vi "String to I16_2.vi"(11 "Test Case In":refnum<class "test Electronic Datasheet.lvclass">) -> (0 "error out":errorcluster, 3 "Test Case Out":refnum<class "test Electronic Datasheet.lvclass">)   [LabVIEW 2024, in "test Electronic Datasheet.lvclass"]
uses:
  test Electronic Datasheet.lvclass
  test Electronic Datasheet.lvclass/test Electronic Datasheet.ctl
  Core/Electronic Datasheet.lvlib
  d54f7c7f-f69a-4a4c-9201-5aaad2364e05.vi
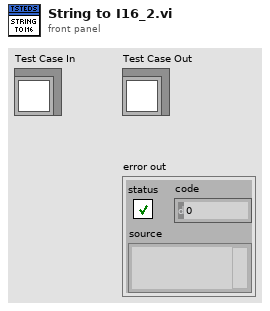
[diagram p1: front panel]
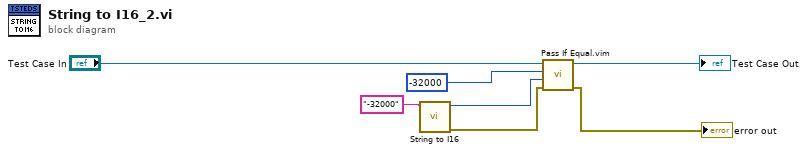
[diagram p0: block diagram]
diagram:
  n1 = call "String to I16.vi"("String"="-32000") -> ("error out"=w3:errorcluster, "I16"=w1:i16)  [unwired: 9 in]
  n2 = call "Pass If Equal.vim"("error in (no error)"=w3, "Actual"=w1, "Expected"=i16 -32000, "LUnit Test Case In"="Test Case In") -> ("error out"=→"error out":errorcluster, "LUnit Test Case Out"=→"Test Case Out":refnum<class "test Electronic Datasheet.lvclass">)  [unwired: 6 in]
